vi "SynchronousPump_OneCommand.vi"(8 "error in (no error)":errorcluster, 9 "Command":string, 10 "Pump #":dbl, 11 "VISA Refnum in":refnum<visa-resource-name>) -> (0 "error out":errorcluster, 1 "EXIT PROGRAM? (F)":bool, 2 "Read (Response)":string, 3 "VISA Refnum out":refnum<visa-resource-name>)   [LabVIEW 2013]
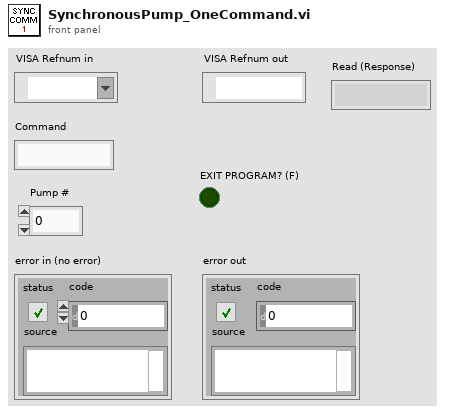
[diagram p1: front panel]
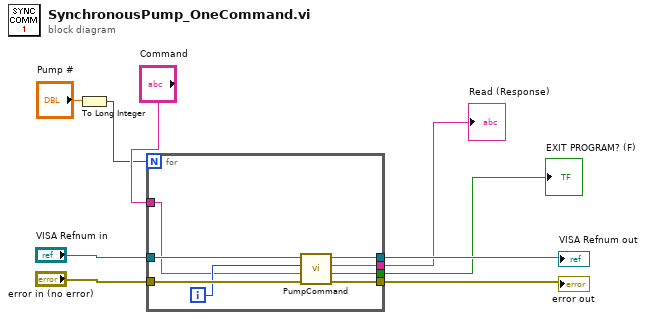
[diagram p0: block diagram]
diagram:
  n1 = To Long Integer(number="Pump #") -> (32bit integer=w3:i32)
  n2 = for {
    N: w3 -> [_]
    tunnel: "VISA Refnum in" -> [w17]
    tunnel: "error in (no error)" -> [w16]
    tunnel: [w14] -> w8
    tunnel: [w13] -> w7
    tunnel: "Command" -> [w12]
    tunnel: [w11] -> w2
    tunnel: [w10] -> w1
    i -> [w15]
    n3 = call "PumpCommand.vi"("error in (no error)"=w16, "Command:"=w12, "Pump Address"=w15, "VISA Refnum in"=w17) -> ("error out"=w14:errorcluster, "EXIT PROGRAM? (F)"=w10:bool, "Read (Response)"=w11:string, "VISA resource name out"=w13:refnum<visa-resource-name>)  [unwired: 3 in]
  }
  "error out" <- w8
  "VISA Refnum out" <- w7
  "Read (Response)" <- w2
  "EXIT PROGRAM? (F)" <- w1
